vi "Get Groups.vi"(8 "error in (no error)":errorcluster, 11 "TDMS Log File Specification in":refnum<class "TDMS Log File Specification.lvclass">) -> (0 "error out":errorcluster, 2 "Groups":T1[](array[typedef]), 3 "TDMS Log File Specification out":refnum<class "TDMS Log File Specification.lvclass">)   [LabVIEW 2015, in "TDMS Log File Specification.lvclass"]
uses:
  TDMS Log File Specification.lvclass
  Channel Group Specification.ctl
  Property Specification.ctl
  Channel Specification.ctl
  TDMS Log File Specification.lvclass/TDMS Log File Specification.ctl
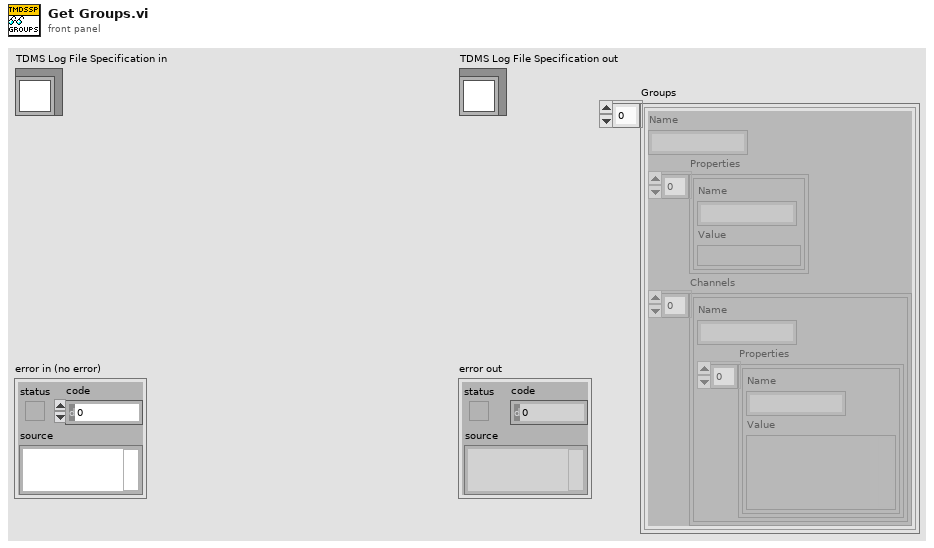
[diagram p1: front panel]
types:
  T1 = typedef "TDMS Log File Specification.lvclass/Channel Group Specification.ctl" = cluster{"Name":string, "Properties":T2[], "Channels":T3[]}
  T2 = typedef "TDMS Log File Specification.lvclass/Property Specification.ctl" = cluster{"Name":string, "Value":variant}
  T3 = typedef "TDMS Log File Specification.lvclass/Channel Specification.ctl" = cluster{"Name":string, "Properties":T2[]}
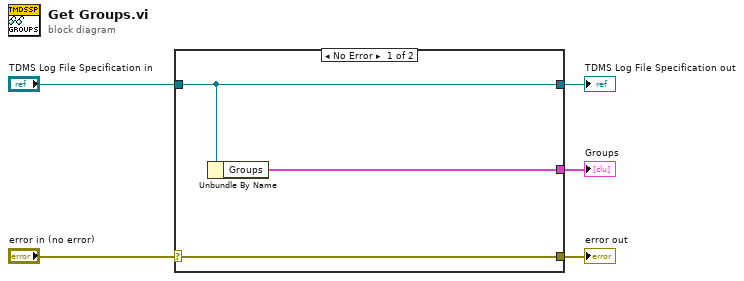
[diagram p0: block diagram]
diagram:
  n1 = case shown="No Error" "error in (no error)" {
    selector: "error in (no error)" -> [w8 w9]
    tunnel: [w8 w9] -> w4
    tunnel: [w7 w10] -> w2
    tunnel: "TDMS Log File Specification in" -> [w7 w10]
    tunnel: [w6 _] -> w1
    frame No Error {
      n2 = Unbundle By Name(w7) -> ("Groups"=w6:T1[])
    }
    frame Error {
    }
  }
  "error out" <- w4
  "TDMS Log File Specification out" <- w2
  "Groups" <- w1
